vi "add_open_brace.vi"(8 "error in (no error)":errorcluster, 11 "Instrument Command In":string) -> (0 "error out":errorcluster, 3 "Instrument Command Out":string)   [LabVIEW 2018]
uses:
  <vilib>/regexp/Match Regular Expression.xnode
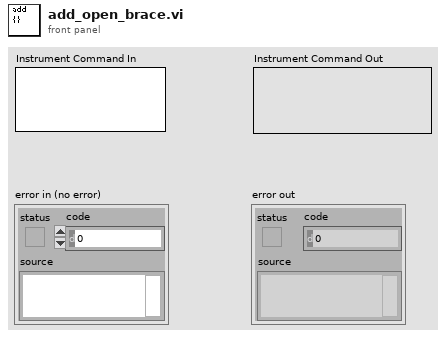
[diagram p1: front panel]
types:
  T1 = cluster{"Start Sting":string, "End String":string}
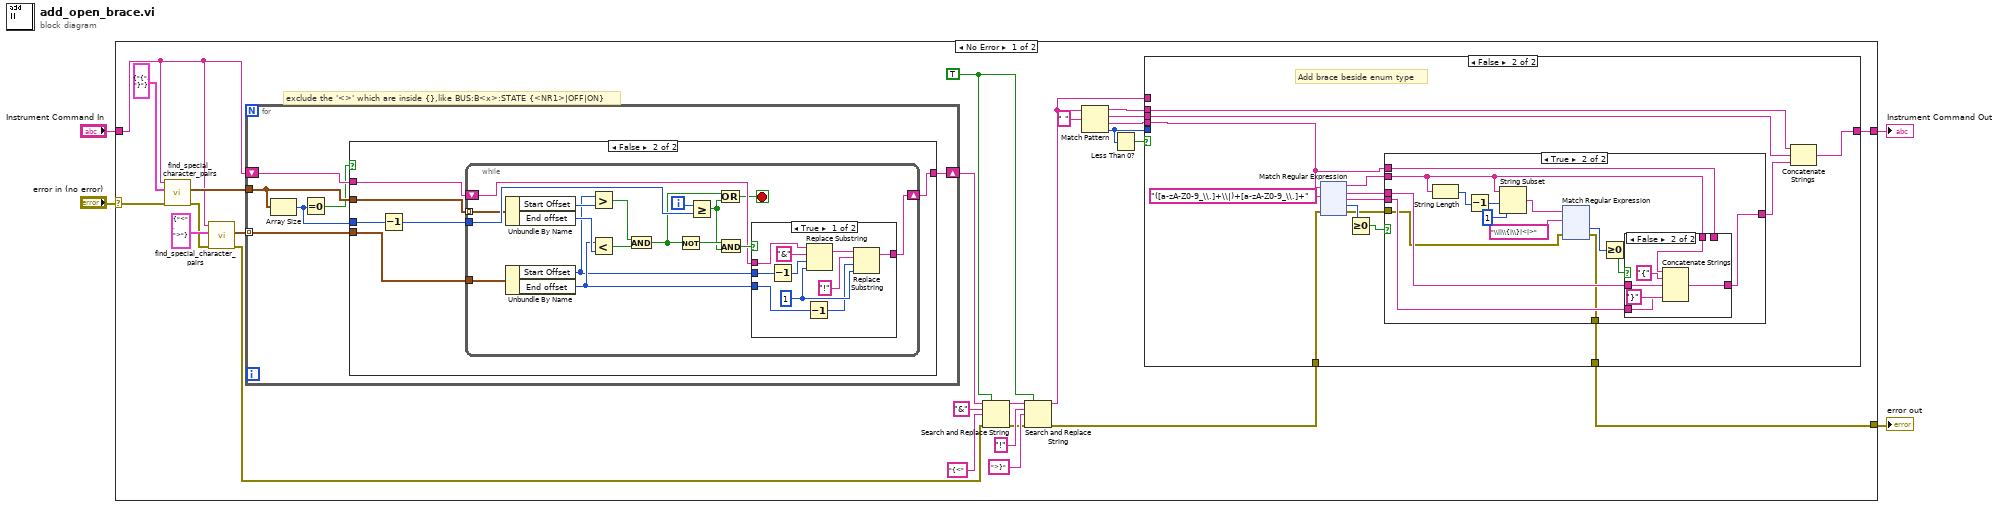
[diagram p0: block diagram]
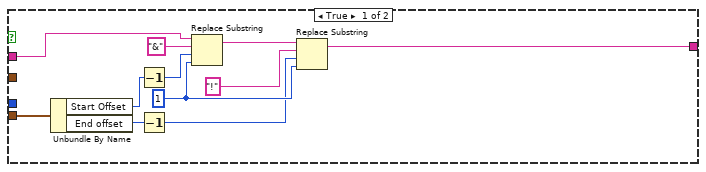
[diagram p5: hidden frame]
diagram:
  n1 = case shown="No Error" "error in (no error)" {
    selector: "error in (no error)" -> [w11 w343]
    tunnel: [w30 w344] -> w4
    tunnel: "Instrument Command In" -> [w14 w344]
    tunnel: [w5 w343] -> w1
    frame No Error {
      w23 = TRUE
      # "exclude the '<>' which are inside {},like BUS:B<x>:STATE {<NR1>|OFF|ON}"
      n2 = call "find_special_character_pairs.vi"("error in (no error)"=w11, "String Pair"=T1 {"Start Sting"="{", "End String"="}"}, "Command String"=w14) -> ("error out"=w10:errorcluster, "Pair Offset"=w17:cluster{"Start Offset":i32, "End offset":i32}[])  [unwired: 7 out]
      n3 = call "find_special_character_pairs.vi"("error in (no error)"=w10, "String Pair"=T1 {"Start Sting"="<", "End String"=">"}, "Command String"=w14) -> ("error out"=w9:errorcluster, "Pair Offset"=w16:cluster{"Start Offset":i32, "End offset":i32}[])  [unwired: 7 out]
      n4 = for {
        tunnel: w16 -> [w297] mode=indexing
        tunnel: w17 -> [w296]
        shift-right: [w295] -> w15
        shift-left: w14 -> [w294]
        n5 = Array Size(array=w296) -> (size(s)=w293:i32)
        n6 = Equal To 0?(x=w293) -> (x = 0?=w292:bool)
        n7 = case shown="False" w292 {
          tunnel: w293 -> [_ w314]
          tunnel: w297 -> [w308 w312]
          tunnel: w296 -> [_ w311]
          tunnel: [w304 w310] -> w295
          tunnel: w294 -> [w305 w309]
          frame True {
            w300 = 1 ("length (len. of substring)")
            n8 = Unbundle By Name(w308) -> ("Start Offset"=w307:i32, "End offset"=w306:i32)
            n9 = Decrement(x=w307) -> (x-1=w299:i32)
            n10 = Decrement(x=w306) -> (x-1=w298:i32)
            n11 = Replace Substring(2:w300, 3:w299, 4:"&" ("substring (\"\")"), 5:w305) -> (1:w302:string)  [unwired: 1 out]
            n12 = Replace Substring(2:w300, 3:w298, 4:"!" ("substring (\"\")"), 5:w302) -> (1:w304:string)  [unwired: 1 out]
          }
          frame False {
            n13 = Decrement(x=w314) -> (x-1=w313:i32)
            n14 = while {
              tunnel: w313 -> [w330]
              tunnel: w312 -> [w320]
              tunnel: w311 -> [w329] mode=indexing
              shift-right: [w316] -> w310
              shift-left: w309 -> [w317]
              i -> [w331]
              stop <- w315 stop-if-true
              n15 = Unbundle By Name(w329) -> ("Start Offset"=w328:i32, "End offset"=w327:i32)
              n16 = Unbundle By Name(w320) -> ("Start Offset"=w318:i32, "End offset"=w319:i32)
              n17 = Greater?(x=w318, y=w328) -> (0:w326:bool)
              n18 = Less?(x=w319, y=w327) -> (x < y?=w325:bool)
              n19 = And(x=w326, y=w325) -> (x .and. y?=w324:bool)
              n20 = Not(x=w324) -> (.not. x?=w323:bool)
              n21 = Greater Or Equal?(x=w331, y=w330) -> (x >= y?=w322:bool)
              n22 = Or(x=w324, y=w322) -> (x .or. y?=w315:bool)
              n23 = And(x=w323, y=w322) -> (x .and. y?=w321:bool)
              n24 = case shown="True" w321 {
                tunnel: w319 -> [w339 _]
                tunnel: w317 -> [w341 w342]
                tunnel: w318 -> [w340 _]
                tunnel: [w336 w342] -> w316
                frame True {
                  w334 = 1 ("length (len. of substring)")
                  n25 = Decrement(x=w340) -> (x-1=w333:i32)
                  n26 = Decrement(x=w339) -> (x-1=w332:i32)
                  n27 = Replace Substring(2:w334, 3:w333, 4:"&" ("substring (\"\")"), 5:w341) -> (1:w337:string)  [unwired: 1 out]
                  n28 = Replace Substring(2:w334, 3:w332, 4:"!" ("substring (\"\")"), 5:w337) -> (1:w336:string)  [unwired: 1 out]
                }
                frame False {
                }
              }
            }
          }
        }
      }
      n29 = Search and Replace String(replace all?=w23, input string=w15, search string="&", replace string="{<" ("replace string (\"\")"), error in=w9) -> (result string=w29:string, error out=w24:errorcluster)  [unwired: 5 out]
      n30 = Search and Replace String(replace all?=w23, input string=w29, search string="!", replace string=">}" ("replace string (\"\")"), error in=w24) -> (result string=w20:string, error out=w6:errorcluster)  [unwired: 5 out]
      n31 = Match Pattern(string=w20, regular expression=" ") -> (before substring=w8:string, match substring=w7:string, after substring=w21:string, offset past match=w13:i32)  [unwired: 1 out]
      n32 = Less Than 0?(x=w13) -> (x < 0?=w12:bool)
      n33 = case shown="False" w12 {
        tunnel: [w32 w46] -> w30
        tunnel: w21 -> [_ w45]
        tunnel: w20 -> [w32 _]
        tunnel: w13 -> [_ _]
        tunnel: w8 -> [_ w44]
        tunnel: w7 -> [_ w43]
        tunnel: w6 -> [w31 w42]
        tunnel: [w31 w41] -> w5
        frame True {
          # "Action-Status CMD"
        }
        frame False {
          # "Add brace beside enum type"
          n34 = xnode "Match Regular Expression"("input string"=w45, "regular expression"="([a-zA-Z0-9_\\.]+\\|)+[a-zA-Z0-9_\\.]+", "error in"=w42) -> ("before match"=w39:string, "whole match"=w38:string, "after match"=w37:string, "offset past match"=w35:i32, "error out"=w33:errorcluster)  [unwired: 1 in, 2 out]
          n35 = Greater Or Equal To 0?(x=w35) -> (x >= 0?=w34:bool)
          n36 = case shown="True" w34 {
            tunnel: w39 -> [w48 w50]
            tunnel: w38 -> [_ w62]
            tunnel: w37 -> [_ w61]
            tunnel: [w48 w60] -> w36
            tunnel: w33 -> [w47 w54]
            tunnel: [w47 w53] -> w41
            tunnel: w45 -> [_ w49]
            frame False {
            }
            frame True {
              n37 = String Length(string=w50) -> (length=w59:i32)
              n38 = Decrement(x=w59) -> (x-1=w58:i32)
              n39 = String Subset(string=w50, offset (0)=w58, length (rest)=1 ("length (rest)")) -> (substring=w56:string)
              n40 = xnode "Match Regular Expression"("input string"=w56, "regular expression"="\\||\\{|\\}|<|>", "error in"=w54) -> ("offset past match"=w52:i32, "error out"=w53:errorcluster)  [unwired: 1 in, 5 out]
              n41 = Greater Or Equal To 0?(x=w52) -> (x >= 0?=w51:bool)
              n42 = case shown="False" w51 {
                tunnel: w62 -> [_ w69]
                tunnel: w61 -> [_ w66]
                tunnel: [w63 w65] -> w60
                tunnel: w50 -> [_ w64]
                tunnel: w49 -> [w63 _]
                frame True {
                }
                frame False {
                  n43 = Concatenate Strings(w64, "{" ("string"), w69, "}" ("string"), w66) -> (w65:string)
                }
              }
            }
          }
          n44 = Concatenate Strings(w44, w43, w36) -> (w46:string)
        }
      }
    }
    frame Error {
    }
  }
  "Instrument Command Out" <- w4
  "error out" <- w1
